vi "Obtain.vi"() -> (0 "error out":errorcluster, 2 "Self Queue":refnum<data-value>)   [LabVIEW 2021, in "jettl.lvlib" / "Self Queue.lvlib"]
uses:
  Self Queue.lvlib
  Msg Strategy/Msg Strategy.lvclass
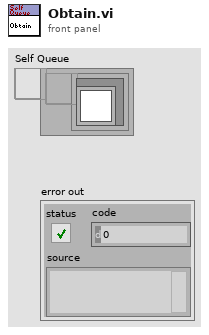
[diagram p1: front panel]
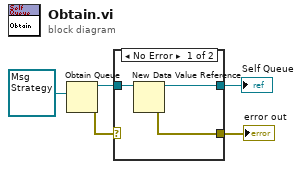
[diagram p0: block diagram]
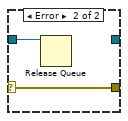
[diagram p2: hidden frame]
diagram:
  n1 = Obtain Queue(element data type=refnum<class "Msg Strategy.lvclass"> refnum ("Msg.lvclass")) -> (queue out=w4:refnum<queue>, error out=w5:errorcluster)  [unwired: 4 in, 1 out]
  n2 = case shown="No Error" w5 {
    selector: w5 -> [_ w9]
    tunnel: w4 -> [w8 w10]
    tunnel: [w7 _] -> w1
    tunnel: [w6 w9] -> w3
    frame No Error {
      n3 = New Data Value Reference(data value=w8) -> (data value reference=w7:refnum<data-value>, error out=w6:errorcluster)  [unwired: 1 in]
    }
    frame Error {
      n4 = Release Queue(queue=w10) -> ()  [unwired: 2 in, 3 out]
    }
  }
  "error out" <- w3
  "Self Queue" <- w1
